vi "lab 2.2.vi"() -> ()   [LabVIEW 2020]
uses:
  <vilib>/measure/madcrms.llb/Basic Averaged DC-RMS for 1 Chan.vi
  <vilib>/measure/NI_MAPro.lvlib
panel:
  out "Array":dbl[](array[numeric])
  out "Numeric 3":dbl
  out "amp 2":dbl
  out "Waveform Graph 3":dynamicdata(graph)
  out "dc":dbl format="%#_64g"
  out "Waveform Graph 2":waveform(dbl)(graph)
  out "Waveform Graph":dynamicdata(graph)
  in  "Offset":dbl
  in  "Amplitude":dbl=1.0
  in  "Frequency":dbl=100.0
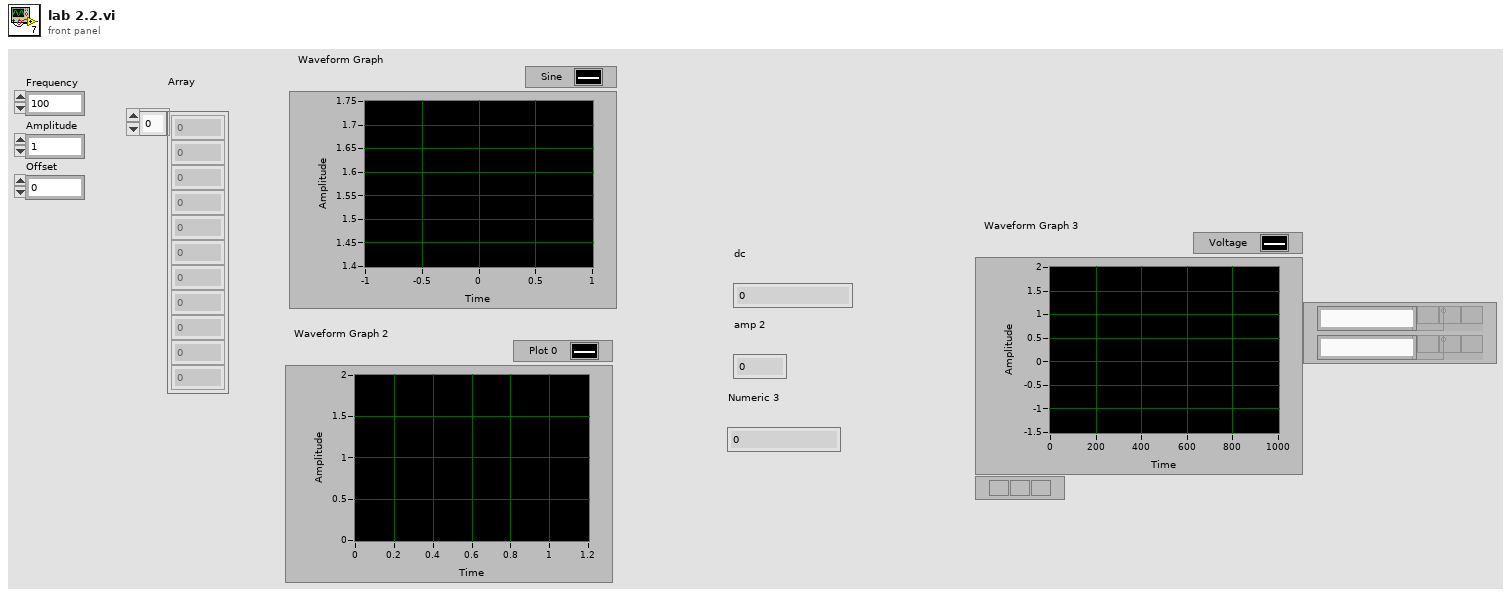
[diagram p1: front panel]
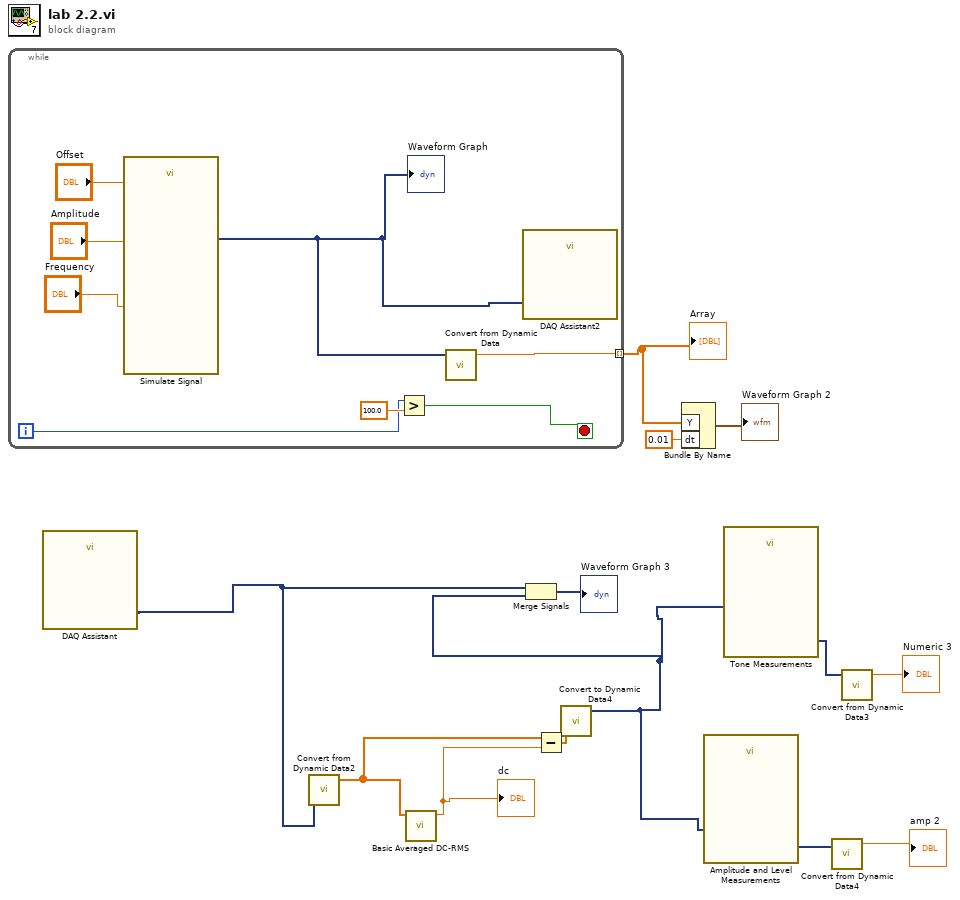
[diagram p0: block diagram]
diagram:
  n1 = while {
    tunnel: [w18] -> w1 mode=indexing
    i -> [w15]
    stop <- w14 stop-if-true
    n2 = call "Simulate Signal"("Offset"="Offset", "Frequency"="Frequency", "Amplitude"="Amplitude") -> ("Sine"=w17:dynamicdata)  [unwired: 11 in, 1 out]
    "Waveform Graph" <- w17
    n3 = Greater?(x=w15, y=100.0) -> (0:w14:bool)
    n4 = call "Convert from Dynamic Data"("Dynamic Data Type"=w17) -> ("Scalar"=w18:dbl)  [unwired: 3 in]
    n5 = call "DAQ Assistant2"("data"=w17) -> ()  [unwired: 17 in, 2 out]
  }
  "Array" <- w1
  n6 = call "DAQ Assistant"() -> ("data"=w5:dynamicdata)  [unwired: 17 in, 2 out]
  n7 = call "Convert from Dynamic Data2"("Dynamic Data Type"=w5) -> ("Array"=w3:dbl[])  [unwired: 3 in]
  n8 = call-poly <vilib>:"Basic Averaged DC-RMS.vi"("signal in"=w3) -> ("DC value"=w11:dbl)  [unwired: 7 in, 3 out]
  "dc" <- w11
  n9 = Subtract(x=w3, y=w11) -> (x-y=w4:dbl[])
  n10 = call "Convert to Dynamic Data4"("Array"=w4) -> ("Dynamic Data Type"=w2:dynamicdata)  [unwired: 3 in]
  n11 = Merge Signals(w5, w2) -> (→"Waveform Graph 3":dynamicdata)
  n12 = Bundle By Name("Y"=w1, "dt"=0.01) -> (→"Waveform Graph 2":waveform(dbl))  [unwired: 1 in]
  n13 = call "Amplitude and Level Measurements"("Signals"=w2) -> ("Peak to Peak"=w6:dynamicdata)  [unwired: 13 in, 1 out]
  n14 = call "Tone Measurements"("Signals"=w2) -> ("Frequency"=w9:dynamicdata)  [unwired: 8 in, 2 out]
  n15 = call "Convert from Dynamic Data4"("Dynamic Data Type"=w6) -> ("Scalar"=→"amp 2":dbl)  [unwired: 3 in]
  n16 = call "Convert from Dynamic Data3"("Dynamic Data Type"=w9) -> ("Scalar"=→"Numeric 3":dbl)  [unwired: 3 in]
